vi "Write Transmission Data Unit.vi"(8 "error in":errorcluster, 10 "transmission data unit":refnum<class "Transmission Data Unit.lvclass">, 11 "Modbus instance in":refnum<class "Modbus API.lvclass">) -> (0 "error out":errorcluster, 3 "Modbus instance out":refnum<class "Modbus API.lvclass">)   [LabVIEW 2021, in "Modbus API.lvclass"]
doc: "This VI is an accessor for the transmission data unit stored in the modbus instance. This accessor can be used as a property node. The transmission data unit is used by the device to determine how to pack and unpack data coming from the physical bus."
uses:
  Modbus API.lvclass
  Modbus API.lvclass/Modbus API.ctl
  Network Protocol/Network Protocol.lvclass
  Transmission Data Unit/Transmission Data Unit.lvclass
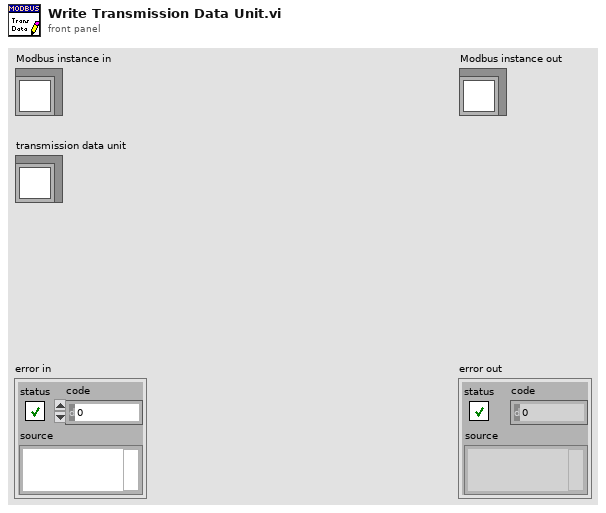
[diagram p1: front panel]
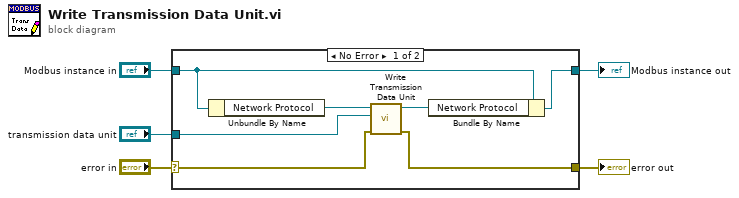
[diagram p0: block diagram]
diagram:
  n1 = case shown="No Error" "error in" {
    selector: "error in" -> [w7 w13]
    tunnel: [w6 w13] -> w4
    tunnel: [w8 w14] -> w2
    tunnel: "Modbus instance in" -> [w11 w14]
    tunnel: "transmission data unit" -> [w12 _]
    frame No Error {
      n2 = Unbundle By Name(w11) -> ("Network Protocol"=w10:refnum<class "Network Protocol.lvclass">)
      n3 = call "Write Transmission Data Unit.vi"("error in (no error)"=w7, "Transmission Data Unit"=w12, "Network Protocol in"=w10) -> ("error out"=w6:errorcluster, "Network Protocol out"=w9:refnum<class "Network Protocol.lvclass">)  [unwired: 7 in]
      n4 = Bundle By Name(cluster=w11, "Network Protocol"=w9) -> (w8:refnum<class "Modbus API.lvclass">)
    }
    frame Error {
    }
  }
  "error out" <- w4
  "Modbus instance out" <- w2
